vi "XNET Signal Property Node.vi"   [LabVIEW 2018]
doc: "Property node used to read/write properties for an XNET Signal I/O name."
uses:
  <resource>/objmgr/xnet.rc
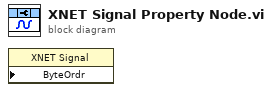
[diagram p0: block diagram]
diagram:
  n1 = property class="XNET Signal" props=["ByteOrdr"]() -> ()  [unwired: 3 in, 2 out]
